vi "Solve PnP (USAC).vi"(6 "Camera Parameters":T7, 7 "USAC Params (Default: OpenCV Defaults) in":refnum<class "USAC Params.lvclass">, 8 "error in (no error)":errorcluster, 11 "Point Correspondence Set":T1) -> (0 "error out":errorcluster, 3 "Pose":T4, 4 "Inliers":i32[](array[numeric]))   [LabVIEW 2020, in "ar.lvlib"]
doc: "Estimate the Pose in the presence of noise or incorrect point correspondences. This function can employ a range of point rejection and pose optimisation methods. \n\nSee https://docs.opencv.org/4.10.0/de/d3e/tutorial_usac.html for more details."
uses:
  ar.lvlib
  common/Camera Parameters.ctl
  common/Camera Matrix.ctl
  common/Camera Distortion Coefficients.ctl
  Pose.ctl
  rvec.ctl
  tvec.ctl
  Point Correspondence Set.ctl
  common/Object Point (Float).ctl
  common/Image Point (Float).ctl
  USAC Params/USAC Params.lvclass
  USAC Params/USAC Params.lvclass/USAC Params.ctl
  common/common.lvlib
  common/bin/gartoolkit_ar_32-1.dll
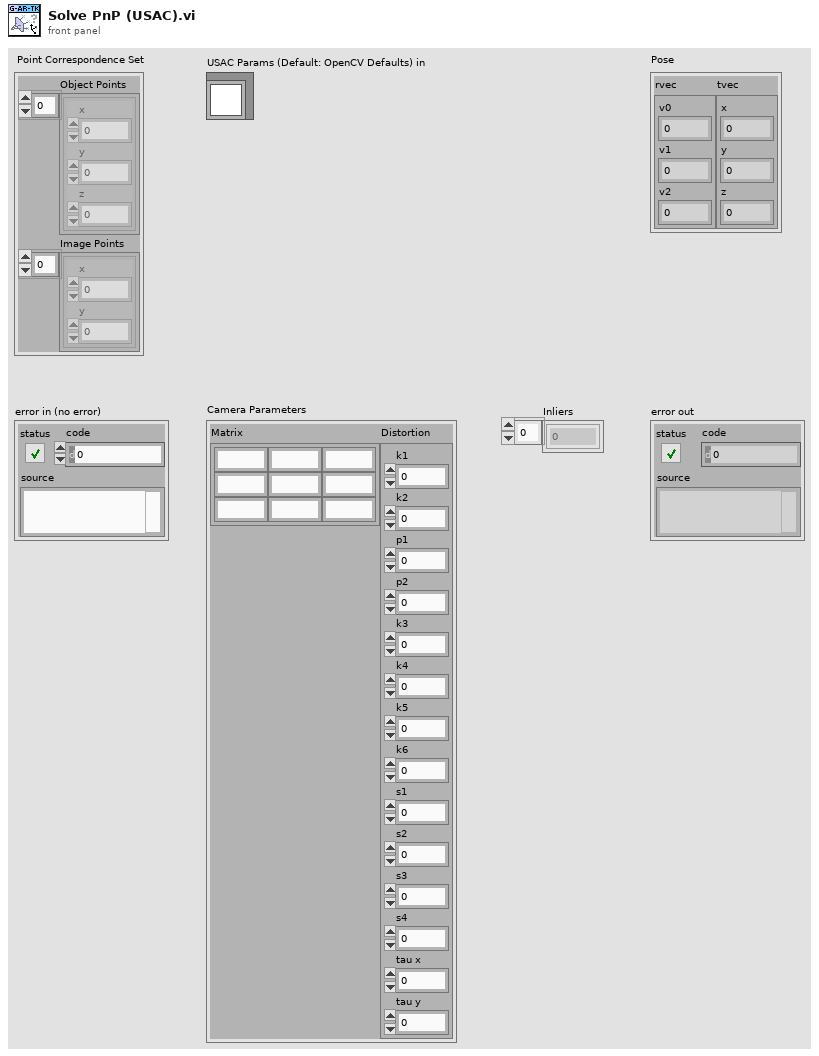
[diagram p1: front panel]
types:
  T1 = typedef "ar.lvlib/Point Correspondence Set.ctl" = cluster{"Object Points":T2[], "Image Points":T3[]}
  T2 = typedef "common.lvlib/Object Point (Float).ctl" = cluster{"x":dbl, "y":dbl, "z":dbl}
  T3 = typedef "common.lvlib/Image Point (Float).ctl" = cluster{"x":dbl, "y":dbl}
  T4 = typedef "ar.lvlib/Pose.ctl" = cluster{"rvec":T5, "tvec":T6}
  T5 = typedef "ar.lvlib/rvec.ctl" = cluster{"v0":dbl, "v1":dbl, "v2":dbl}
  T6 = typedef "ar.lvlib/tvec.ctl" = cluster{"x":dbl, "y":dbl, "z":dbl}
  T7 = typedef "common.lvlib/Camera Parameters.ctl" = cluster{"Matrix":T8, "Distortion":T9}
  T8 = typedef "common.lvlib/Camera Matrix.ctl" = cluster{"m 0,0":dbl, "m 0,1":dbl, "m 0,2":dbl, "m 1,0":dbl, "m 1,1":dbl, "m 1,2":dbl, "m 2,0":dbl, "m 2,1":dbl, "m 2,2":dbl}
  T9 = typedef "common.lvlib/Camera Distortion Coefficients.ctl" = cluster{"k1":dbl, "k2":dbl, "p1":dbl, "p2":dbl, "k3":dbl, "k4":dbl, "k5":dbl, "k6":dbl, "s1":dbl, "s2":dbl, "s3":dbl, "s4":dbl, "tau x":dbl, "tau y":dbl}
  T10 = typedef "ar.lvlib/USAC Params.lvclass/Parameters.ctl" = cluster{"Confidence":dbl, "Threshold":dbl, "Final Polisher Iterations":u16, "Local Optimization Iterations":u16, "Local Optimization Sample Size":u16, "Max Iterations":u16, "Random Generator State":i32, "Final Polisher":T11, "Local Optimization Method":T12, "Neighbor Search Method":T13, "Sampler":T14, "Score":T15, "Is Parallel":bool}
  T11 = typedef "ar.lvlib/USAC Params.lvclass/Polishing Methods.ctl" = enum8{"NONE", "LSQ", "MAGSAC", "COV"}
  T12 = typedef "ar.lvlib/USAC Params.lvclass/Local Optimization Methods.ctl" = enum8{"NULL", "INNER_LO", "INNER_AND_ITER_LO", "GC", "SIGMA"}
  T13 = typedef "ar.lvlib/USAC Params.lvclass/Neighbor Search Methods.ctl" = enum8{"FLANN_KNN", "GRID", "FLANN_RADIUS"}
  T14 = typedef "ar.lvlib/USAC Params.lvclass/Sampling Methods.ctl" = enum8{"UNIFORM", "PROGRESSIVE_NAPSAC", "NAPSAC", "PROSAC"}
  T15 = typedef "ar.lvlib/USAC Params.lvclass/Score Methods.ctl" = enum8{"RANSAC", "MSAC", "MAGSAC", "LMEDS"}
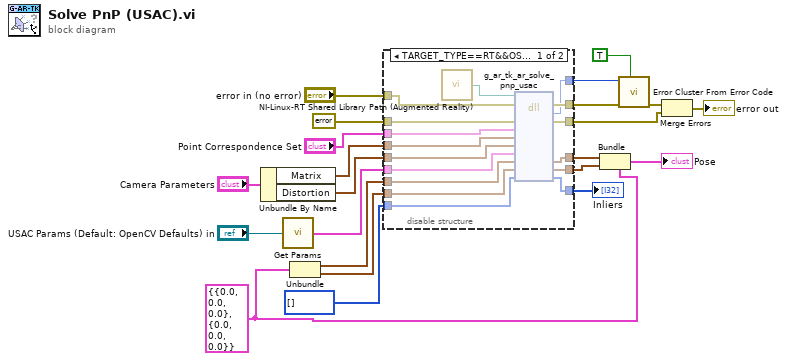
[diagram p0: block diagram]
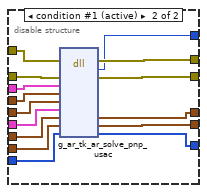
[diagram p2: hidden frame]
diagram:
  w20 = T4 {"rvec"={"v0"=0.0, "v1"=0.0, "v2"=0.0}, "tvec"={"x"=0.0, "y"=0.0, "z"=0.0}} ("Pose (Estimate)")
  n1 = Unbundle By Name("Camera Parameters") -> ("Matrix"=w13:T8, "Distortion"=w12:T9)
  n2 = call "Get Params.vi"("USAC Params in"="USAC Params (Default: OpenCV Defaults) in") -> ("Parameters"=w11:T10)
  n3 = Unbundle(w20) -> ("rvec"=w10:T5, "tvec"=w9:T6)
  n4 = disable-structure shown="TARGET_TYPE==RT&&OS==Linux" {
    disable-tunnel: "error in (no error)" -> [w38 w53]
    disable-tunnel: errorcluster {"status"=FALSE, "code"=0, "source"=""} ("error constant") -> [w37 w52]
    disable-tunnel: "Point Correspondence Set" -> [w36 w51]
    disable-tunnel: w13 -> [w35 w50]
    disable-tunnel: w12 -> [w34 w49]
    disable-tunnel: w11 -> [w33 w48]
    disable-tunnel: w10 -> [w32 w47]
    disable-tunnel: w9 -> [w31 w46]
    disable-tunnel: i32[] [] ("inliers") -> [w30 w45]
    disable-tunnel: [w29 w44] -> w7
    disable-tunnel: [w28 w43] -> w6
    disable-tunnel: [w27 w42] -> w5
    disable-tunnel: [w26 w41] -> w4
    disable-tunnel: [w25 w40] -> w3
    disable-tunnel: [w24 w39] -> w2
    frame condition #0 {
      n5 = call "NI-Linux-RT Shared Library Path (Augmented Reality).vi"() -> ("Path"=w23:path)
      n6 = dll-call lib="?" fn="g_ar_tk_ar_solve_pnp_usac" ("g_ar_toolkit.*.*:g_ar_tk_image_copy")(path in=w23, error in=w38, "error_cluster"=w37, "corespondence"=w36, "camera_matrix"=w35, "camera_distortion"=w34, "usac_parameters"=w33, "rvec"=w32, "tvec"=w31, "inliers"=w30) -> (error out=w29:errorcluster, w28:i32, "error_cluster"=w27:errorcluster, "rvec"=w26:T5, "tvec"=w25:T6, "inliers"=w24:i32[])  [unwired: 5 in, 1 out]
    }
    frame condition #1 (active) {
      n7 = dll-call lib="C:/serenial/lib/g-augmented-reality-toolkit/LabVIEW/common/bin/gartoolkit_ar_*-1.*" fn="g_ar_tk_ar_solve_pnp_usac" ("g_ar_toolkit.*.*:g_ar_tk_image_copy")(error in=w53, "error_cluster"=w52, "corespondence"=w51, "camera_matrix"=w50, "camera_distortion"=w49, "usac_parameters"=w48, "rvec"=w47, "tvec"=w46, "inliers"=w45) -> (error out=w44:errorcluster, w43:i32, "error_cluster"=w42:errorcluster, "rvec"=w41:T5, "tvec"=w40:T6, "inliers"=w39:i32[])  [unwired: 6 in, 1 out]
    }
  }
  "Inliers" <- w2
  n8 = Bundle(cluster=w20, "rvec"=w4, "tvec"=w3) -> (→"Pose":T4)
  n9 = call <vilib>:"Error Cluster From Error Code.vi"("show call chain? (False)"=TRUE, "error in (no error)"=w7, "error code (0)"=w6) -> ("error out"=w18:errorcluster)  [unwired: 6 in]
  n10 = Merge Errors(w18, w5) -> (→"error out":errorcluster)
